vi "Calculate_checksum.vi"(1 "Data":i32[](array[numeric]) format="%.0x") -> (0 "Checksum":i32)   [LabVIEW 2019]
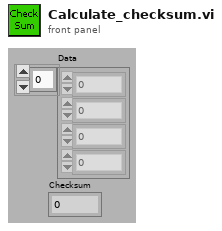
[diagram p1: front panel]
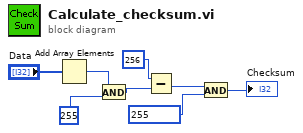
[diagram p0: block diagram]
diagram:
  n1 = Add Array Elements(numeric array="Data") -> (sum=w8:i32)
  n2 = And(x=w8, y=255) -> (x .and. y?=w5:i32)
  n3 = Subtract(x=256, y=w5) -> (x-y=w3:i32)
  n4 = And(x=w3, y=255) -> (x .and. y?=→"Checksum":i32)
